vi "Station_Coordinates.vi"() -> ()   [LabVIEW 2012]
panel:
  out "Station altitude":dbl
  out "Station longitude":dbl
  out "Station latitude":dbl
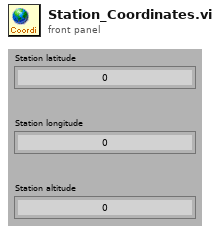
[diagram p1: front panel]
diagram:
